vi "EminemTeleop.vi"(8 "CmdCancel":bool, 9 "CmdPreRev":bool, 10 "CmdAmpDeliver":bool, 11 "CmdShoot":bool) -> ()   [LabVIEW 2023]
doc: "Makes sure the actual position of the arm is within 5 degrees of the setpoint/target"
uses:
  <vilib>/Rock Robotics/WPI/ThirdParty/JAS_Junk/TrajLib/Trajectory_Library.lvlib
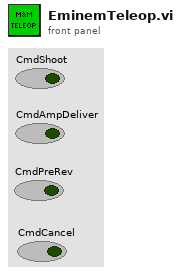
[diagram p1: front panel]
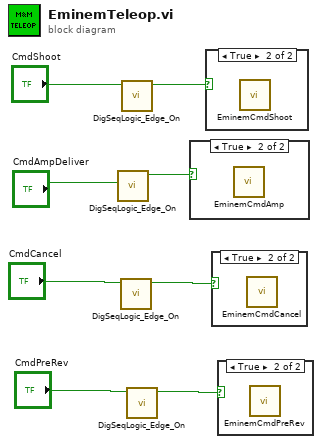
[diagram p0: block diagram]
diagram:
  n1 = call <vilib>:"DigSeqLogic_Edge_On.vi"("Input"="CmdAmpDeliver") -> ("On Edge"=w8:bool)  [unwired: 10 in]
  n2 = call <vilib>:"DigSeqLogic_Edge_On.vi"("Input"="CmdCancel") -> ("On Edge"=w3:bool)  [unwired: 10 in]
  n3 = call <vilib>:"DigSeqLogic_Edge_On.vi"("Input"="CmdShoot") -> ("On Edge"=w7:bool)  [unwired: 10 in]
  n4 = call <vilib>:"DigSeqLogic_Edge_On.vi"("Input"="CmdPreRev") -> ("On Edge"=w1:bool)  [unwired: 10 in]
  n5 = case shown="True" w8 {
    frame False {
    }
    frame True {
      n6 = call "EminemCmdAmp.vi"() -> ()  [unwired: 12 in]
    }
  }
  n7 = case shown="True" w7 {
    frame False {
    }
    frame True {
      n8 = call "EminemCmdShoot.vi"() -> ()  [unwired: 11 in, 1 out]
    }
  }
  n9 = case shown="True" w3 {
    frame False {
    }
    frame True {
      n10 = call "EminemCmdCancel.vi"() -> ()  [unwired: 12 in]
    }
  }
  n11 = case shown="True" w1 {
    frame False {
    }
    frame True {
      n12 = call "EminemCmdPreRev.vi"() -> ()  [unwired: 11 in, 1 out]
    }
  }
